vi "Jaguar Drive Distance Sync.vi"(8 "error in (no error)":errorcluster, 10 "Rotations":dbl=2.0, 11 "RobotDriveDevRef":T1) -> (0 "error out":errorcluster, 3 "RobotDriveDevRef Out":T1)   [LabVIEW 2013]
uses:
  <vilib>/Rock Robotics/WPI/RobotDrive/WPI_RobotDriveDevRef.ctl
  <vilib>/Rock Robotics/WPI/MotorControl/WPI_MotorControlDeviceRef.ctl
  <vilib>/Rock Robotics/SystemInterfaces/Typedef/FPGA_TypedefDigitalModule.ctl
  <vilib>/Rock Robotics/SystemInterfaces/DIO/FPGA_DIOPWMChannel.ctl
  <vilib>/Rock Robotics/WPI/PWM/WPI_PWMDeadband.ctl
  <vilib>/Rock Robotics/WPI/CAN/Jaguar/SubVIs/WPI_CANJaguar_ControlMode.ctl
  <vilib>/Rock Robotics/WPI/PWM/WPI_PWMTransform_ConPane.ctl
  <vilib>/Rock Robotics/WPI/CAN/Jaguar/SubVIs/WPI_CANJaguar_StatusSelect.ctl
panel:
  in  "Setteling Ticks":i32=10
  in  "Target V Range":dbl=0.008
  out "Encoder Output":cluster{"Position":dbl, "Position":dbl}(graph)
  out "Right Motor Output":T9(graph)
  out "Left Motor Output":T9(graph)
  out "Exec Time":u32(graph)
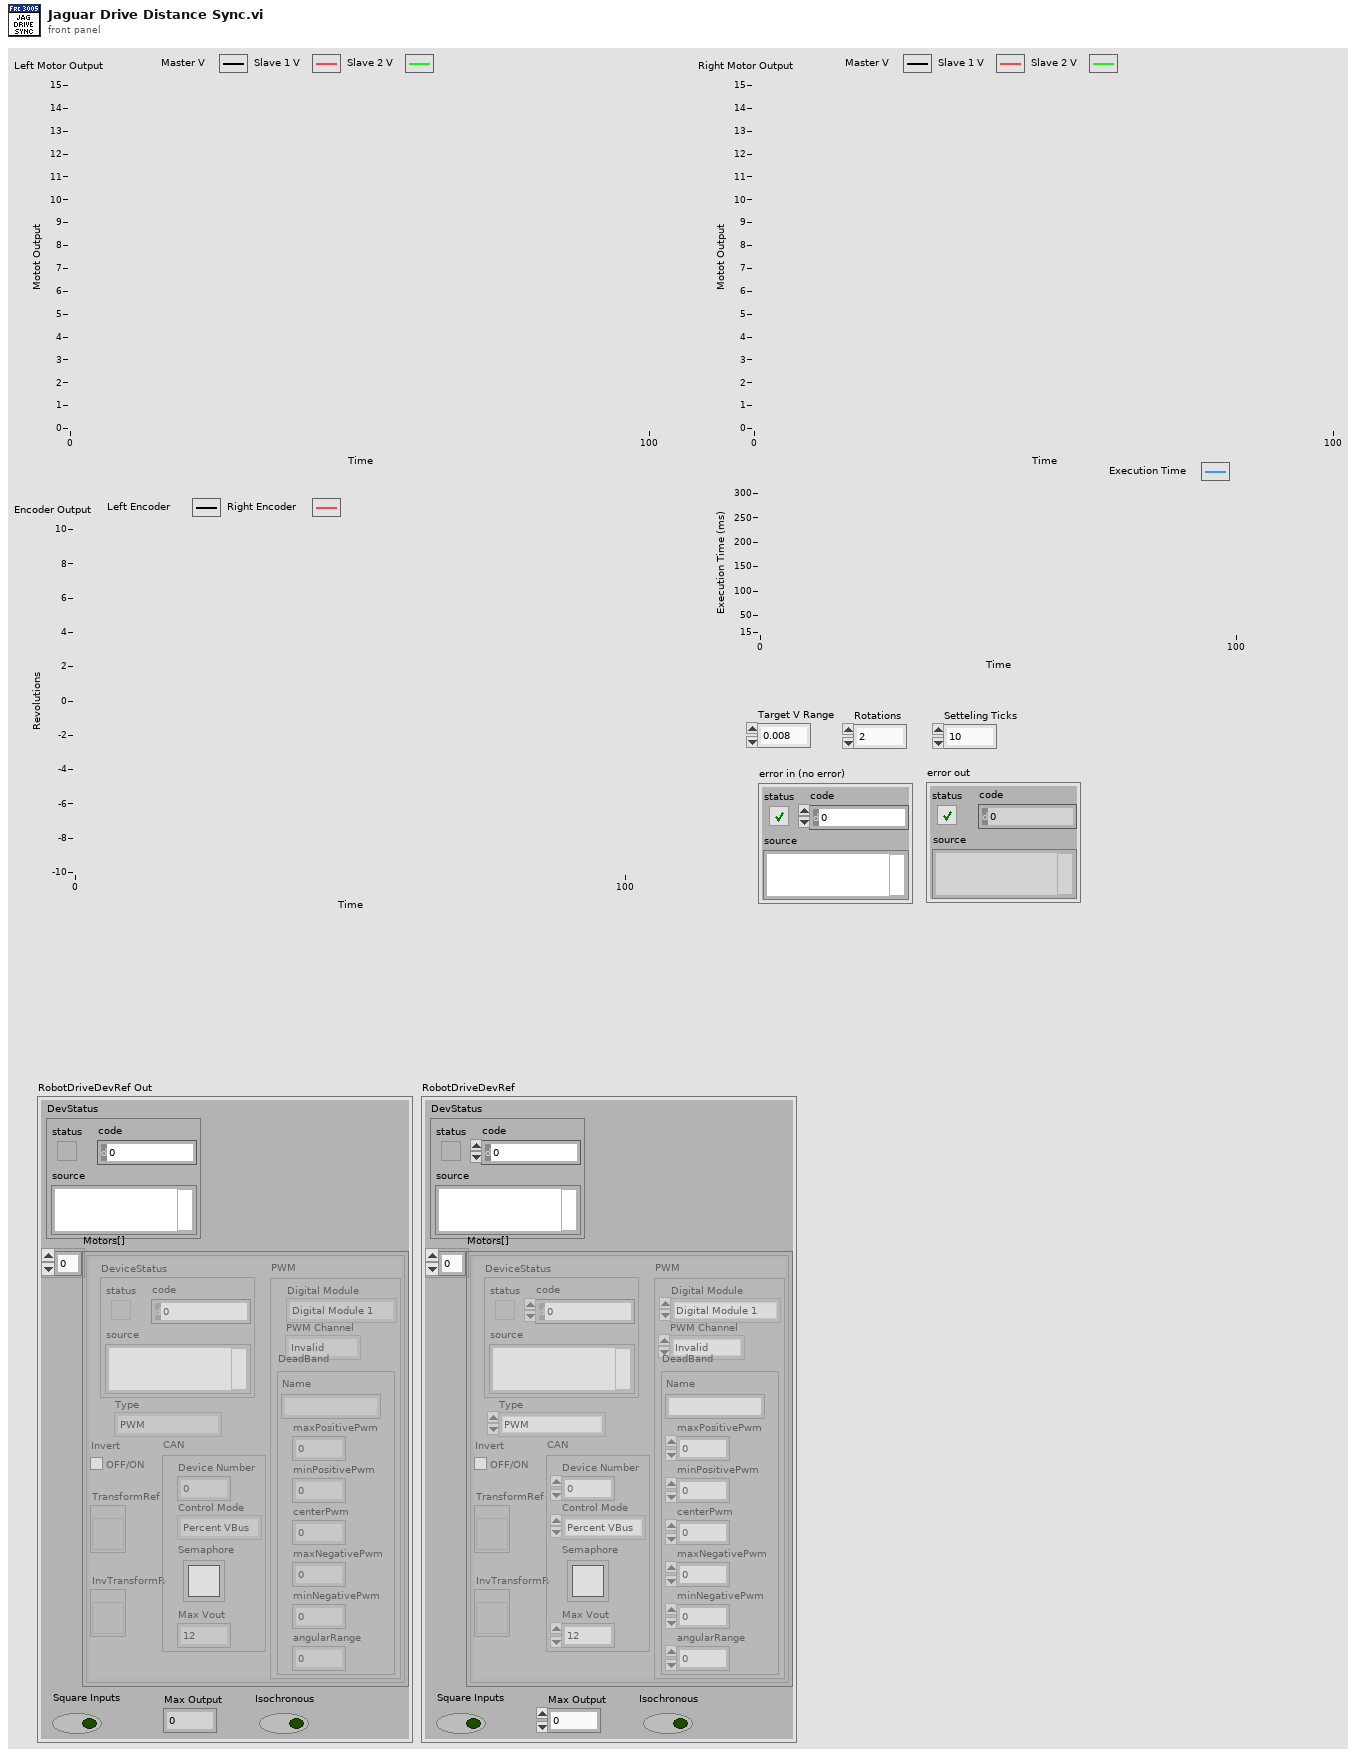
[diagram p1: front panel]
types:
  T1 = typedef "WPI_RobotDriveDevRef.ctl" = cluster{"DevStatus":errorcluster, "Motors[]":T2[], "Square Inputs":bool, "Max Output":dbl, "Isochronous":bool}
  T2 = typedef "WPI_MotorControlDeviceRef.ctl" = cluster{"DeviceStatus":errorcluster, "Type":enum16{"PWM", "CAN"}, "PWM":cluster{"Digital Module":T3, "PWM Channel":T4, "DeadBand":T5}, "CAN":cluster{"Device Number":u8, "Control Mode":T6, "Semaphore":T7, "Max Vout":dbl}, "Invert":bool, "TransformRef":T8, "InvTransformRef":T8}
  T3 = typedef "FPGA_TypedefDigitalModule.ctl" = enum16{"Digital Module 1", "Digital Module 2"}
  T4 = typedef "FPGA_DIOPWMChannel.ctl" = enum8{"PWM 1", "PWM 2", "PWM 3", "PWM 4", "PWM 5", "PWM 6", "PWM 7", "PWM 8", "PWM 9", "PWM 10", "Invalid"}
  T5 = typedef "WPI_PWMDeadband.ctl" = cluster{"Name":string, "maxPositivePwm":i32, "minPositivePwm":i32, "centerPwm":i32, "maxNegativePwm":i32, "minNegativePwm":i32, "angularRange":u16}
  T6 = typedef "WPI_CANJaguar_ControlMode.ctl" = enum8{"Percent VBus", "Current", "Speed", "Position", "Voltage"}
  T7 = typedef "Semaphore RefNum" = refnum<k1>
  T8 = typedef "WPI_PWMTransform_ConPane.ctl" = refnum<vi>
  T9 = cluster{"Output Voltage":dbl, "Output Voltage":dbl, "Output Voltage":dbl}
  T10 = typedef "WPI_CANJaguar_StatusSelect.ctl" = enum16{"Output Percent VBus", "Output Voltage", "Bus Voltage", "Current", "Temperature", "Position", "Speed", "Limit Switches", "Faults", "Fault Counters", "Power Cycle"}
  T11 = typedef "WPI_CANJaguar_Status.ctl" = cluster{"Output Percent VBus":dbl, "Output Voltage":dbl, "Bus Voltage":dbl, "Current":dbl, "Temperature":dbl, "Position":dbl, "Speed":dbl, "Limits":cluster{"Forward Limit":bool, "Reverse Limit":bool, "Forward Soft Limit":bool, "Reverse Soft Limit":bool, "Sticky Forward Limit":bool, "Sticky Reverse Limit":bool, "Sticky Forward Soft Limit":bool, "Sticky Reverse Soft Limit":bool}, "Faults":cluster{"Current Fault":bool, "Temperature Fault":bool, "Bus Voltage Fault":bool, "Gate Driver Fault":bool, "Comm Fault":bool}, "Fault Counters":cluster{"Current Faults":u8, "Temperature Faults":u8, "Bus Voltage Faults":u8, "Gate Driver Faults":u8, "Comm Faults":u8, "CAN Status":u8, "CAN RX Errors":u8, "CAN TX Errors":u8}, "Power Cycle":bool}
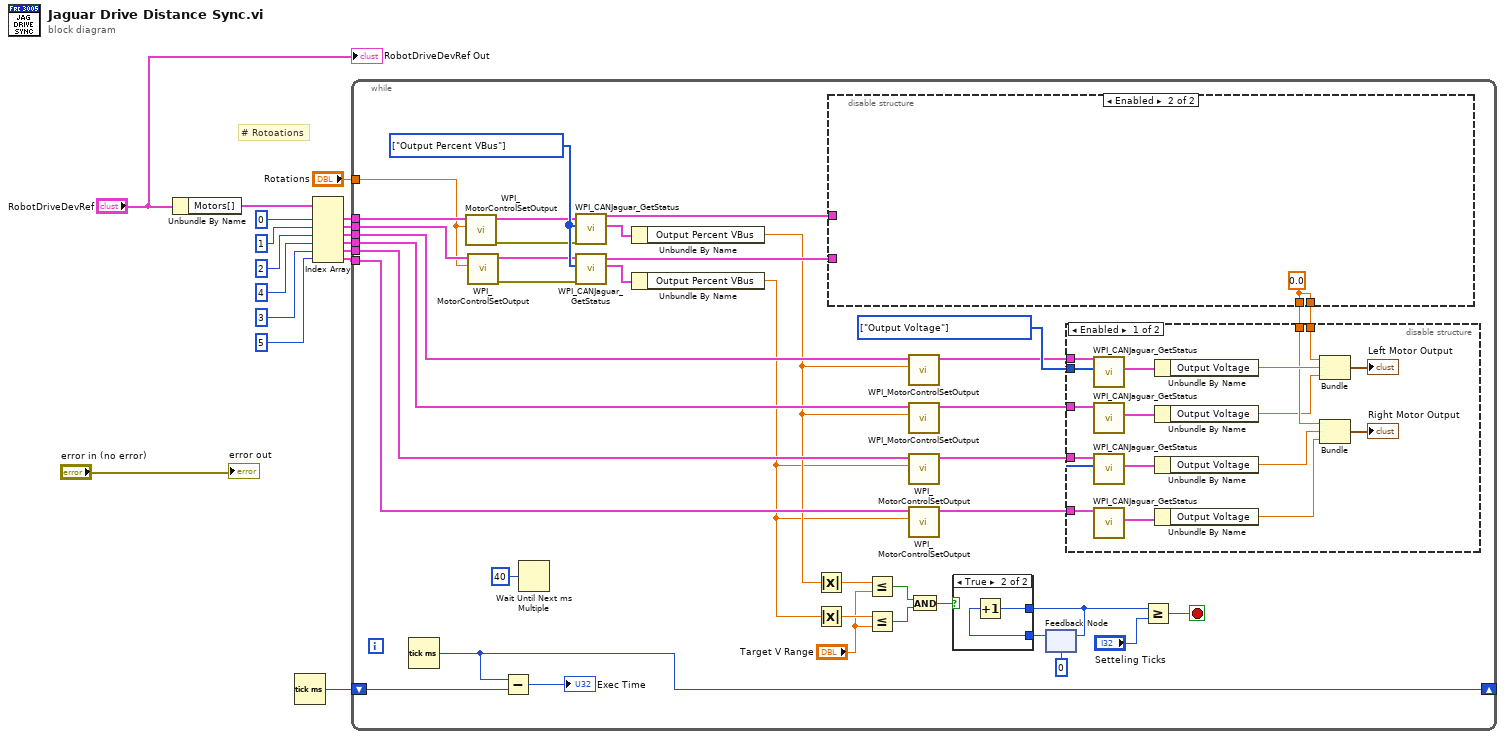
[diagram p0: block diagram]
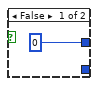
[diagram p2: hidden frame]
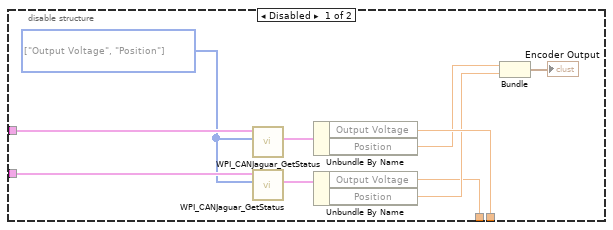
[diagram p4: hidden frame]
diagram:
  # "# Rotoations"
  n1 = Unbundle By Name("RobotDriveDevRef") -> ("Motors[]"=w16:T2[])
  n2 = Tick Count (ms)() -> (millisecond timer value=w3:u32)
  n3 = Index Array(array=w16, index #1=0 ("index"), index #2=1 ("index"), index #3=2 ("index"), index #4=4 ("index"), index #5=3 ("index"), index #6=5 ("index")) -> (element #1=w13:T2, element #2=w12:T2, element #3=w10:T2, element #4=w14:T2, element #5=w11:T2, element #6=w15:T2)
  n4 = while {
    shift-right: [w52] -> _
    shift-left: w3 -> [w53]
    tunnel: w13 -> [w41]
    tunnel: w12 -> [w38]
    tunnel: w10 -> [w44]
    tunnel: w11 -> [w43]
    tunnel: w14 -> [w35]
    tunnel: w15 -> [w34]
    tunnel: "Rotations" -> [w31]
    stop <- w20 stop-if-true
    w49 = T10[] [enum."Output Voltage"] items=["Output Percent VBus", "Output Voltage", "Bus Voltage", "Current", "Temperature", "Position", "Speed", "Limit Switches", "Faults", "Fault Counters", "Power Cycle"] ("Status Select")
    w57 = T10[] [enum."Output Percent VBus"] items=["Output Percent VBus", "Output Voltage", "Bus Voltage", "Current", "Temperature", "Position", "Speed", "Limit Switches", "Faults", "Fault Counters", "Power Cycle"] ("Status Select")
    n5 = Tick Count (ms)() -> (millisecond timer value=w52:u32)
    n6 = call <vilib>:"WPI_MotorControlSetOutput.vi"("Output"=w31, "MotorControlDevRef"=w41) -> ("error out"=w37:errorcluster, "MotorControlDevRef"=w40:T2)  [unwired: 7 in, 1 out]
    n7 = call <vilib>:"WPI_MotorControlSetOutput.vi"("Output"=w31, "MotorControlDevRef"=w38) -> ("error out"=w36:errorcluster, "MotorControlDevRef"=w39:T2)  [unwired: 7 in, 1 out]
    n8 = Subtract(x=w52, y=w53) -> (x-y=→"Exec Time":u32)
    n9 = Wait Until Next ms Multiple(millisecond multiple=u32 40) -> ()  [unwired: 1 out]
    n10 = call <vilib>:"WPI_CANJaguar_GetStatus.vi"("error in (no error)"=w37, "Status Select"=w57, "CAN Jaguar Ref"=w40) -> ("Status"=w55:T11, "CAN Jaguar Ref Out"=w45:T2)  [unwired: 6 in, 1 out]
    n11 = call <vilib>:"WPI_CANJaguar_GetStatus.vi"("error in (no error)"=w36, "Status Select"=w57, "CAN Jaguar Ref"=w39) -> ("Status"=w54:T11, "CAN Jaguar Ref Out"=w46:T2)  [unwired: 6 in, 1 out]
    n12 = Unbundle By Name(w55) -> ("Output Percent VBus"=w30:dbl)
    n13 = Unbundle By Name(w54) -> ("Output Percent VBus"=w29:dbl)
    n14 = Absolute Value(x=w30) -> (abs(x)=w28:dbl)
    n15 = Absolute Value(x=w29) -> (abs(x)=w27:dbl)
    n16 = disable-structure shown="Enabled" {
      disable-tunnel: [w87 w88] -> w50
      disable-tunnel: w46 -> [w86 _]
      disable-tunnel: w45 -> [w85 _]
      disable-tunnel: [w81 w88] -> w42
      frame Disabled {
        w80 = T10[] [enum."Output Voltage", enum."Position"] items=["Output Percent VBus", "Output Voltage", "Bus Voltage", "Current", "Temperature", "Position", "Speed", "Limit Switches", "Faults", "Fault Counters", "Power Cycle"] ("Status Select")
        n17 = call <vilib>:"WPI_CANJaguar_GetStatus.vi"("Status Select"=w80, "CAN Jaguar Ref"=w85) -> ("Status"=w79:T11)  [unwired: 7 in, 2 out]
        n18 = call <vilib>:"WPI_CANJaguar_GetStatus.vi"("Status Select"=w80, "CAN Jaguar Ref"=w86) -> ("Status"=w78:T11)  [unwired: 7 in, 2 out]
        n19 = Unbundle By Name(w79) -> ("Output Voltage"=w87:dbl, "Position"=w84:dbl)
        n20 = Unbundle By Name(w78) -> ("Output Voltage"=w81:dbl, "Position"=w83:dbl)
        n21 = Bundle("Position"=w84, "Position"=w83) -> (→"Encoder Output":cluster{"Position":dbl, "Position":dbl})  [unwired: 1 in]
      }
      frame Enabled {
        w88 = 0.0 ("Output Voltage")
      }
    }
    n22 = Less Or Equal?(x=w28, y="Target V Range") -> (x <= y?=w25:bool)
    n23 = Less Or Equal?(x=w27, y="Target V Range") -> (x <= y?=w24:bool)
    n24 = call <vilib>:"WPI_MotorControlSetOutput.vi"("Output"=w30, "MotorControlDevRef"=w44) -> ("MotorControlDevRef"=w47:T2)  [unwired: 7 in, 2 out]
    n25 = call <vilib>:"WPI_MotorControlSetOutput.vi"("Output"=w30, "MotorControlDevRef"=w35) -> ("MotorControlDevRef"=w32:T2)  [unwired: 7 in, 2 out]
    n26 = call <vilib>:"WPI_MotorControlSetOutput.vi"("Output"=w29, "MotorControlDevRef"=w43) -> ("MotorControlDevRef"=w48:T2)  [unwired: 7 in, 2 out]
    n27 = call <vilib>:"WPI_MotorControlSetOutput.vi"("Output"=w29, "MotorControlDevRef"=w34) -> ("MotorControlDevRef"=w33:T2)  [unwired: 7 in, 2 out]
    n28 = And(x=w25, y=w24) -> (x .and. y?=w23:bool)
    n29 = feedback #1(0) -> (w22:i32)
    n30 = case shown="True" w23 {
      tunnel: [0 w59] -> w19
      tunnel: w22 -> [_ w60]
      frame False {
      }
      frame True {
        n31 = Increment(x=w60) -> (x+1=w59:i32)
      }
    }
    n32 = feedback-in #1(w19) -> ()
    n33 = disable-structure shown="Enabled" {
      disable-tunnel: w50 -> [w77 _]
      disable-tunnel: w49 -> [w74 _]
      disable-tunnel: w48 -> [w73 _]
      disable-tunnel: w47 -> [w72 _]
      disable-tunnel: w42 -> [w71 _]
      disable-tunnel: w33 -> [w68 _]
      disable-tunnel: w32 -> [w67 _]
      frame Enabled {
        n34 = call <vilib>:"WPI_CANJaguar_GetStatus.vi"("Status Select"=w74, "CAN Jaguar Ref"=w72) -> ("Status"=w64:T11)  [unwired: 7 in, 2 out]
        n35 = call <vilib>:"WPI_CANJaguar_GetStatus.vi"("CAN Jaguar Ref"=w67) -> ("Status"=w61:T11)  [unwired: 8 in, 2 out]
        n36 = call <vilib>:"WPI_CANJaguar_GetStatus.vi"("Status Select"=w74, "CAN Jaguar Ref"=w73) -> ("Status"=w63:T11)  [unwired: 7 in, 2 out]
        n37 = call <vilib>:"WPI_CANJaguar_GetStatus.vi"("CAN Jaguar Ref"=w68) -> ("Status"=w62:T11)  [unwired: 8 in, 2 out]
        n38 = Unbundle By Name(w64) -> ("Output Voltage"=w76:dbl)
        n39 = Unbundle By Name(w61) -> ("Output Voltage"=w66:dbl)
        n40 = Unbundle By Name(w63) -> ("Output Voltage"=w75:dbl)
        n41 = Unbundle By Name(w62) -> ("Output Voltage"=w65:dbl)
        n42 = Bundle("Output Voltage"=w77, "Output Voltage"=w76, "Output Voltage"=w66) -> (→"Left Motor Output":T9)  [unwired: 1 in]
        n43 = Bundle("Output Voltage"=w71, "Output Voltage"=w75, "Output Voltage"=w65) -> (→"Right Motor Output":T9)  [unwired: 1 in]
      }
      frame Disabled {
      }
    }
    n44 = Greater Or Equal?(x=w19, y="Setteling Ticks") -> (x >= y?=w20:bool)
  }
  "error out" <- "error in (no error)"
  "RobotDriveDevRef Out" <- "RobotDriveDevRef"
